vi "Get DataArray (String).vi"(8 "error in (no error)":errorcluster, 11 "DataTable in":refnum<class "DataTable.lvclass">) -> (0 "error out":errorcluster, 2 "Array":string[][](array[string]), 3 "DataTable out":refnum<class "DataTable.lvclass">)   [LabVIEW 2016, in "DataGrid.lvlib" / "DataTable.lvclass"]
uses:
  <userlib>/LabVIEWdotNetDataGrid/source/DataTable/DataTable.lvclass
  <userlib>/LabVIEWdotNetDataGrid/source/DataTable/DataTable.lvclass/DataTable.ctl
  System.Data
  <userlib>/LabVIEWdotNetDataGrid/source/GridColumn/GridColumn.lvclass/GridColumn.ctl
  <userlib>/LabVIEWdotNetDataGrid/source/GridColumn/Read datatype.vi
  <userlib>/LabVIEWdotNetDataGrid/source/GridColumn/GridColumn.lvclass
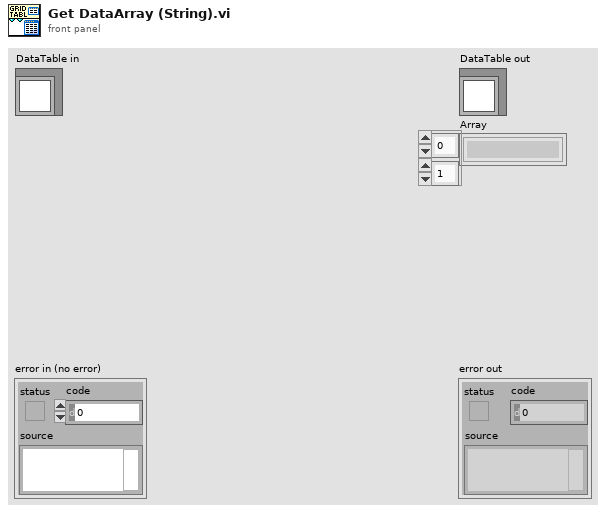
[diagram p1: front panel]
types:
  T1 = typedef "DataGrid.lvlib/GridColumn.lvclass/ColumnType.ctl" = enum16{"string", "image", "check", "numeric", "timestamp", "button", "combo", "link"}
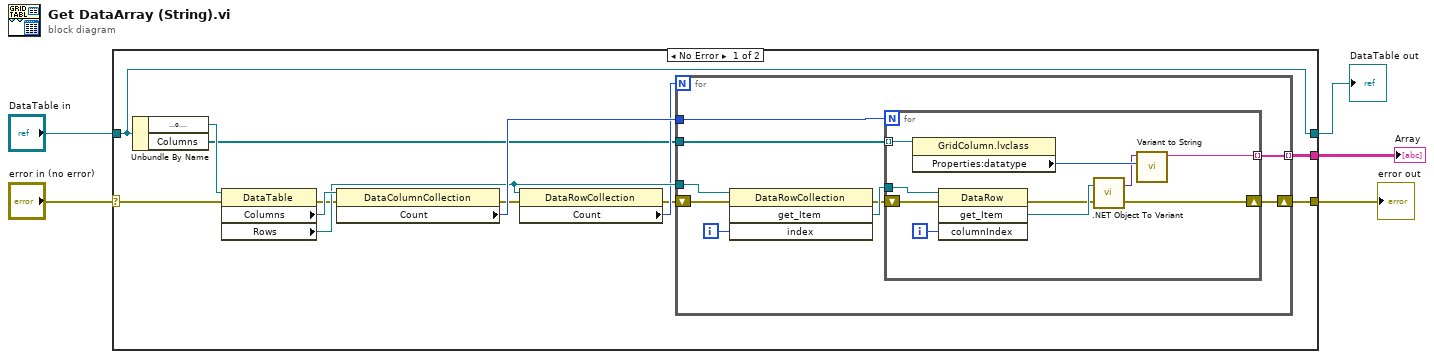
[diagram p0: block diagram]
diagram:
  n1 = case shown="No Error" "error in (no error)" {
    selector: "error in (no error)" -> [w11 w38]
    tunnel: [w10 w38] -> w4
    tunnel: [w18 w39] -> w2
    tunnel: "DataTable in" -> [w18 w39]
    tunnel: [w6 _] -> w1
    frame No Error {
      n2 = Unbundle By Name(w18) -> ("DataTable"=w17:refnum<k24>, "Columns"=w7:refnum<class "GridColumn.lvclass">[])
      n3 = property class="DataTable"(reference=w17, error in=w11) -> (error out=w12:errorcluster, "Columns"=w16:refnum<k24>, "Rows"=w14:refnum<k24>)  [unwired: 1 out]
      n4 = property class="DataColumnCollection"(reference=w16, error in=w12) -> (error out=w9:errorcluster, "Count"=w15:i32)  [unwired: 1 out]
      n5 = property class="DataRowCollection"(reference=w14, error in=w9) -> (error out=w8:errorcluster, "Count"=w13:i32)  [unwired: 1 out]
      n6 = for {
        N: w13 -> [_]
        tunnel: w15 -> [w27]
        tunnel: w14 -> [w26]
        shift-right: [w23] -> w10
        shift-left: w8 -> [w22]
        tunnel: w7 -> [w20]
        tunnel: [w19] -> w6 mode=indexing
        i -> [w25]
        n7 = invoke class="DataRowCollection" method="get_Item"(reference=w26, error in=w22, "index"=w25) -> (error out=w21:errorcluster, "get_Item"=w24:refnum<k24>)  [unwired: 1 in, 2 out]
        n8 = for {
          N: w27 -> [_]
          tunnel: w24 -> [w37]
          shift-right: [w32] -> w23
          shift-left: w21 -> [w35]
          tunnel: w20 -> [w31] mode=indexing
          tunnel: [w28] -> w19 mode=indexing
          i -> [w36]
          n9 = property class="GridColumn.lvclass"(reference=w31) -> ("Properties:datatype"=w30:T1)  [unwired: 1 in, 2 out]
          n10 = invoke class="DataRow" method="get_Item"(reference=w37, error in=w35, "columnIndex"=w36) -> (error out=w33:errorcluster, "get_Item"=w34:refnum<k24>)  [unwired: 1 in, 2 out]
          n11 = call <vilib>:".NET Object To Variant.vi"("error in (no error)"=w33, ".NET object"=w34) -> ("error out"=w32:errorcluster, "variant"=w29:variant)
          n12 = call <userlib>:"Variant to String.vi"("datatype"=w30, "Variant"=w29) -> ("String"=w28:string)  [unwired: 8 in, 1 out]
        }
      }
    }
    frame Error {
    }
  }
  "error out" <- w4
  "DataTable out" <- w2
  "Array" <- w1
